vi "FTW-JSON-Object-SetElement-DBL.vi"(0 "JSON":T1, 5 "Key":string, 7 "Value":dbl, 11 "error in":errorcluster) -> (4 "JSON out":T1, 15 "error out":errorcluster)   [LabVIEW 2015]
uses:
  core/type/FTW-Type-JSON.ctl
panel:
  # "Inputs"
  # "Outputs"
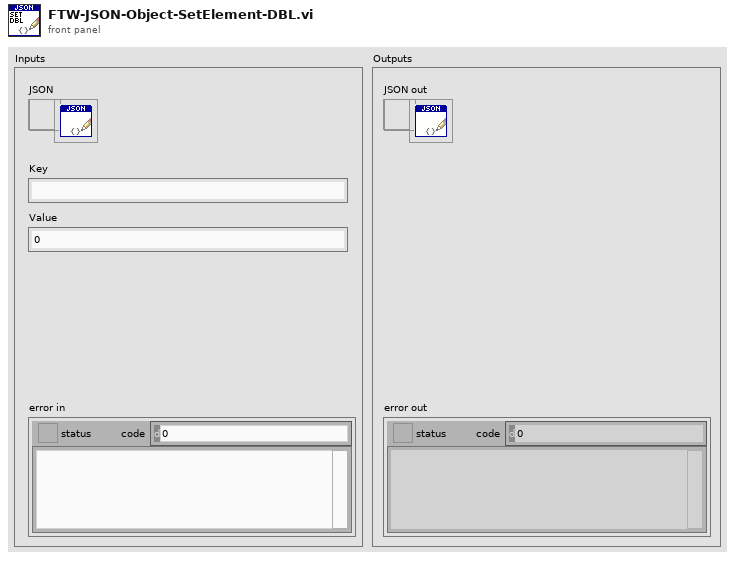
[diagram p1: front panel]
types:
  T1 = typedef "FTW-Type-JSON.ctl" = refnum<data-value>
  T2 = cluster{"FTW-CodeGen-Type":enum16{"FTW-JSON"}, "Object":i64, "EncodingFlags":i64, "DecodingFlags":i64}
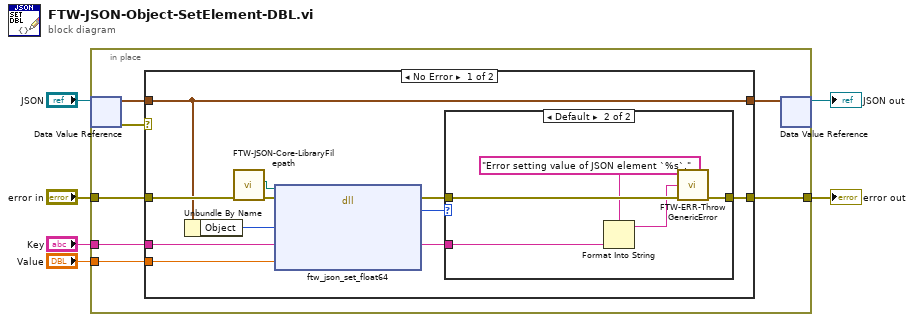
[diagram p0: block diagram]
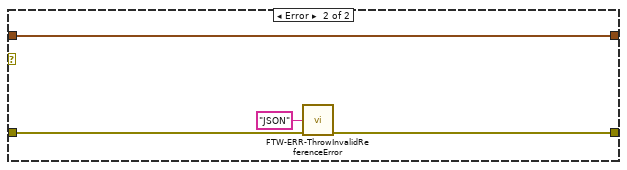
[diagram p3: hidden frame]
diagram:
  n1 = in-place {
    in-place-border: "error in" -> [w9]
    in-place-border: [w10] -> w4
    in-place-border: "Key" -> [w13]
    in-place-border: "Value" -> [w11]
    n2 = in-place-dvr #1("JSON") -> (w12:T2, w8:errorcluster)
    n3 = case shown="No Error" w8 {
      tunnel: w13 -> [w24 _]
      tunnel: w12 -> [w14 w31]
      tunnel: w11 -> [w22 _]
      tunnel: [w18 w32] -> w10
      tunnel: w9 -> [w17 w33]
      tunnel: [w14 w31] -> w7
      frame No Error {
        n4 = Unbundle By Name(w14) -> ("Object"=w23:i64)
        n5 = call "FTW-JSON-Core-LibraryFilepath.vi"("error in"=w17) -> ("error out"=w16:errorcluster, "JSON Library Filepath"=w15:path)  [unwired: 9 in]
        n6 = dll-call lib="?" fn="ftw_json_set_float64"(path in=w15, error in=w16, "JSON Object Pointer"=w23, "Key"=w24, "New Value"=w22) -> (error out=w20:errorcluster, "Return Value"=w21:i64, "Key"=w19:string)  [unwired: 3 in, 1 out]
        n7 = case shown="Default" w21 {
          tunnel: w20 -> [w25 w30]
          tunnel: w19 -> [_ w27]
          tunnel: [w25 w29] -> w18
          frame 0 {
          }
          frame Default {
            n8 = Format Into String(format string="Error setting value of JSON element `%s`.", w27) -> (resulting string=w26:string)  [unwired: 2 in, 1 out]
            n9 = call "FTW-ERR-ThrowGenericError.vi"("Error Message"=w26, "error in"=w30) -> ("error out"=w29:errorcluster)  [unwired: 13 in]
          }
        }
      }
      frame Error {
        n10 = call "FTW-ERR-ThrowInvalidReferenceError.vi"("Reference Type"="JSON", "error in"=w33) -> ("error out"=w32:errorcluster)  [unwired: 13 in]
      }
    }
    n11 = in-place-dvr #1(w7) -> (→"JSON out":T1)  [unwired: 1 out]
  }
  "error out" <- w4
